vi "Init HTTP Server.vi"(8 "error in (no error)":errorcluster, 11 "Vecto in":refnum<class "Vecto.lvclass">) -> (0 "error out":errorcluster, 3 "Vecto out":refnum<class "Vecto.lvclass">)   [LabVIEW 2020, in "Vecto.lvlib" / "Vecto.lvclass"]
uses:
  Vecto.lvclass
  Vecto.lvclass/Vecto.ctl
  lv-http-server/HTTP Server/Server/Server.lvclass
  Node Config/Node Config.lvclass
  Event Level.ctl
  Vecto.lvlib
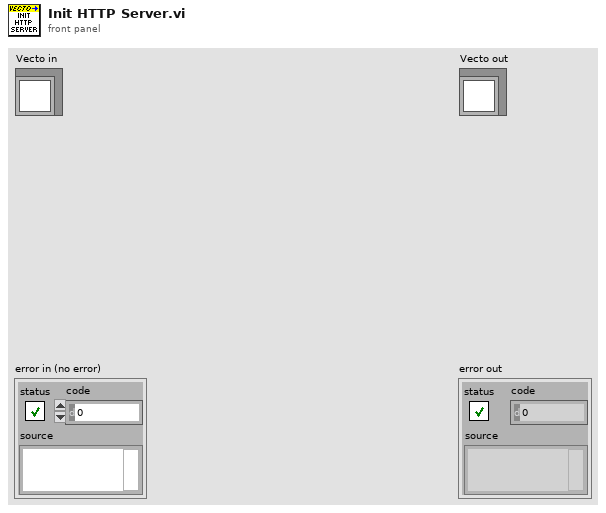
[diagram p1: front panel]
types:
  T1 = typedef "Vecto.lvlib/Event Level.ctl" = enum16{"Debug", "Info", "Warning", "Error"}
  T2 = typedef "Vecto.lvlib/Node Config.lvclass/HTTP Server Info.ctl" = cluster{"HTTP Port":u16, "Debug":bool}
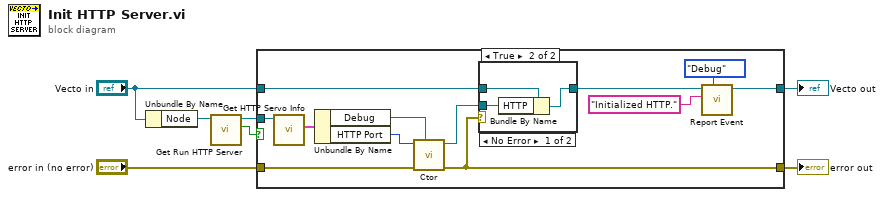
[diagram p0: block diagram]
diagram:
  n1 = Unbundle By Name("Vecto in") -> ("Node"=w7:refnum<class "Node Config.lvclass">)
  n2 = call "Get Run HTTP Server.vi"("Node Config in"=w7) -> ("Run HTTP Server"=w1:bool, "Node Config out"=w2:refnum<class "Node Config.lvclass">)  [unwired: 8 in, 1 out]
  n3 = case shown="True" w1 {
    tunnel: "Vecto in" -> [w9 w21]
    tunnel: "error in (no error)" -> [w8 w19]
    tunnel: [w8 w13] -> w4
    tunnel: [w9 w12] -> w3
    tunnel: w2 -> [_ w17]
    frame False {
    }
    frame True {
      n4 = call "Get HTTP Servo Info.vi"("Node in"=w17) -> ("HTTP Server Info"=w16:T2)  [unwired: 8 in, 2 out]
      n5 = Unbundle By Name(w16) -> ("Debug"=w14:bool, "HTTP Port"=w15:u16)
      n6 = call "Ctor.vi"("Debug (F)"=w14, "error in (no error)"=w19, "HTTP Port (80)"=w15) -> ("error out"=w13:errorcluster, "Server out"=w20:refnum<class "Server.lvclass">)  [unwired: 7 in]
      n7 = case shown="No Error" w13 {
        tunnel: w21 -> [w24 w25]
        tunnel: w20 -> [w23 _]
        tunnel: [w22 w25] -> w18
        frame No Error {
          n8 = Bundle By Name(cluster=w24, "HTTP"=w23) -> (w22:refnum<class "Vecto.lvclass">)
        }
        frame Error {
        }
      }
      n9 = call "Report Event.vi"("Event Level (Info)"=Event_Level."Debug", "Message"="Initialized HTTP.", "Vecto in"=w18) -> ("Vecto out"=w12:refnum<class "Vecto.lvclass">)  [unwired: 7 in, 1 out]
    }
  }
  "error out" <- w4
  "Vecto out" <- w3
